vi "Get Custom Device Name.vi"() -> (3 "CD Name":string)   [LabVIEW 2026, in "Template Engine.lvlib"]
uses:
  Template Engine.lvlib
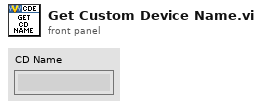
[diagram p1: front panel]
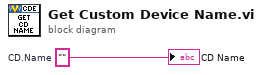
[diagram p0: block diagram]
diagram:
  w1 = ""  # CD.Name
  "CD Name" <- w1
